vi "Create System Control.vi"(8 "error in (no error)":errorcluster, 11 "Device Item Ref in":T1 format="%.0x") -> (0 "error out":errorcluster)   [LabVIEW 2020, in "G5 Regatron Custom Device System Explorer.lvlib"]
uses:
  G5 Regatron Custom Device System Explorer.lvlib
  <vilib>/NI VeriStand/Custom Device API/Custom Device Channel Type.ctl
  <vilib>/NI VeriStand/Custom Device API/Custom Device API.lvlib
  <vilib>/NI VeriStand/Custom Device API/Custom Device Channel.ctl
  <vilib>/NI VeriStand/Custom Device API/Custom Device Item Ref.ctl
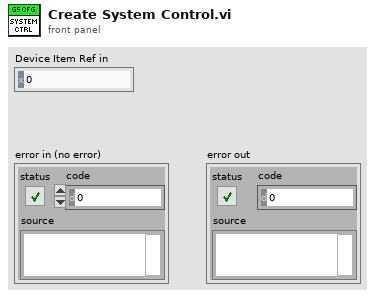
[diagram p1: front panel]
types:
  T1 = typedef "Custom Device API.lvlib/Custom Device Item Ref.ctl" = u64
  T2 = typedef "Custom Device API.lvlib/Custom Device Channel.ctl" = cluster{"Type":T3, "Units":string, "Default Value":dbl, "Faultable":bool, "Scalable":bool}
  T3 = typedef "Custom Device API.lvlib/Custom Device Channel Type.ctl" = enum16{"Input", "Output"}
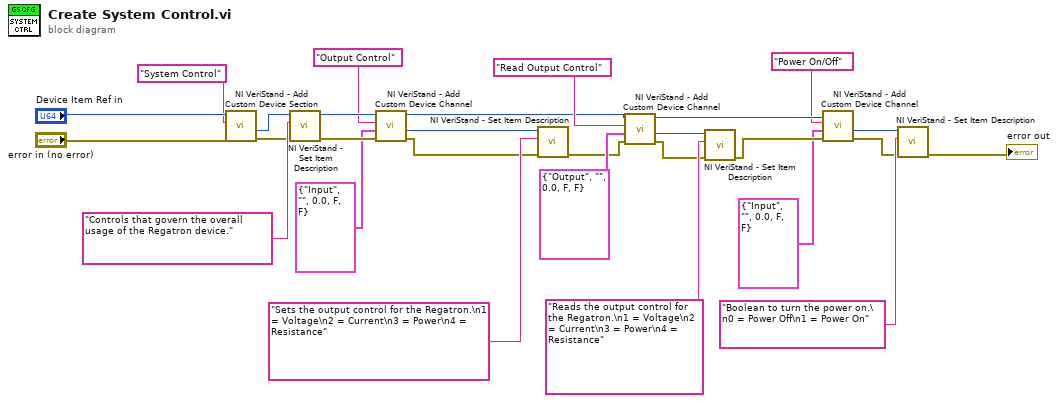
[diagram p0: block diagram]
diagram:
  n1 = call <vilib>:"NI VeriStand - Add Custom Device Section.vi"("error in (no error)"="error in (no error)", "Section Name"="System Control", "Parent Ref in"="Device Item Ref in") -> ("error out"=w13:errorcluster, "Section Ptr"=w15:T1)  [unwired: 5 in, 2 out]
  n2 = call <vilib>:"NI VeriStand - Set Item Description.vi"("error in (no error)"=w13, "Description"="Controls that govern the overall usage of the Regatron device.", "Item Ref in"=w15) -> ("error out"=w14:errorcluster, "Item Ref out"=w16:T1)  [unwired: 6 in, 1 out]
  n3 = call <vilib>:"NI VeriStand - Add Custom Device Channel.vi"("error in (no error)"=w14, "Channel"=T2 {"Type"=enum."Input", "Units"="", "Default Value"=0.0, "Faultable"=FALSE, "Scalable"=FALSE}, "Channel Name"="Output Control", "Parent Ref in"=w16) -> ("error out"=w8:errorcluster, "Channel Ref"=w7:T1, "Parent Ref out"=w20:T1)  [unwired: 4 in, 1 out]
  n4 = call <vilib>:"NI VeriStand - Set Item Description.vi"("error in (no error)"=w8, "Description"="Sets the output control for the Regatron.\n1 = Voltage\n2 = Current\n3 = Power\n4 = Resistance", "Item Ref in"=w7) -> ("error out"=w22:errorcluster)  [unwired: 6 in, 2 out]
  n5 = call <vilib>:"NI VeriStand - Add Custom Device Channel.vi"("error in (no error)"=w22, "Channel"=T2 {"Type"=enum."Output", "Units"="", "Default Value"=0.0, "Faultable"=FALSE, "Scalable"=FALSE}, "Channel Name"="Read Output Control", "Parent Ref in"=w20) -> ("error out"=w25:errorcluster, "Channel Ref"=w24:T1, "Parent Ref out"=w21:T1)  [unwired: 4 in, 1 out]
  n6 = call <vilib>:"NI VeriStand - Set Item Description.vi"("error in (no error)"=w25, "Description"="Reads the output control for the Regatron.\n1 = Voltage\n2 = Current\n3 = Power\n4 = Resistance", "Item Ref in"=w24) -> ("error out"=w26:errorcluster)  [unwired: 6 in, 2 out]
  n7 = call <vilib>:"NI VeriStand - Add Custom Device Channel.vi"("error in (no error)"=w26, "Channel"=T2 {"Type"=enum."Input", "Units"="", "Default Value"=0.0, "Faultable"=FALSE, "Scalable"=FALSE}, "Channel Name"="Power On/Off", "Parent Ref in"=w21) -> ("error out"=w10:errorcluster, "Channel Ref"=w11:T1)  [unwired: 4 in, 2 out]
  n8 = call <vilib>:"NI VeriStand - Set Item Description.vi"("error in (no error)"=w10, "Description"="Boolean to turn the power on.\n0 = Power Off\n1 = Power On", "Item Ref in"=w11) -> ("error out"=→"error out":errorcluster)  [unwired: 6 in, 2 out]
